vi "GetTests.vi"(8 "error in (no error)":errorcluster, 11 "reference in":refnum<class "MES_Local.lvclass">) -> (0 "error out":errorcluster, 1 "Active Test Index":i32, 2 "Tests":T1[](array[typedef]), 3 "reference in":refnum<class "MES_Local.lvclass">)   [LabVIEW 2022 SP3, in "MES_Local.lvlib" / "MES_Local.lvclass"]
uses:
  MES_Local.lvclass
  Components/MES_Base.lvlibp/Controls/Test.ctl
  Components/MES_Base.lvlibp/MES_Base.lvclass
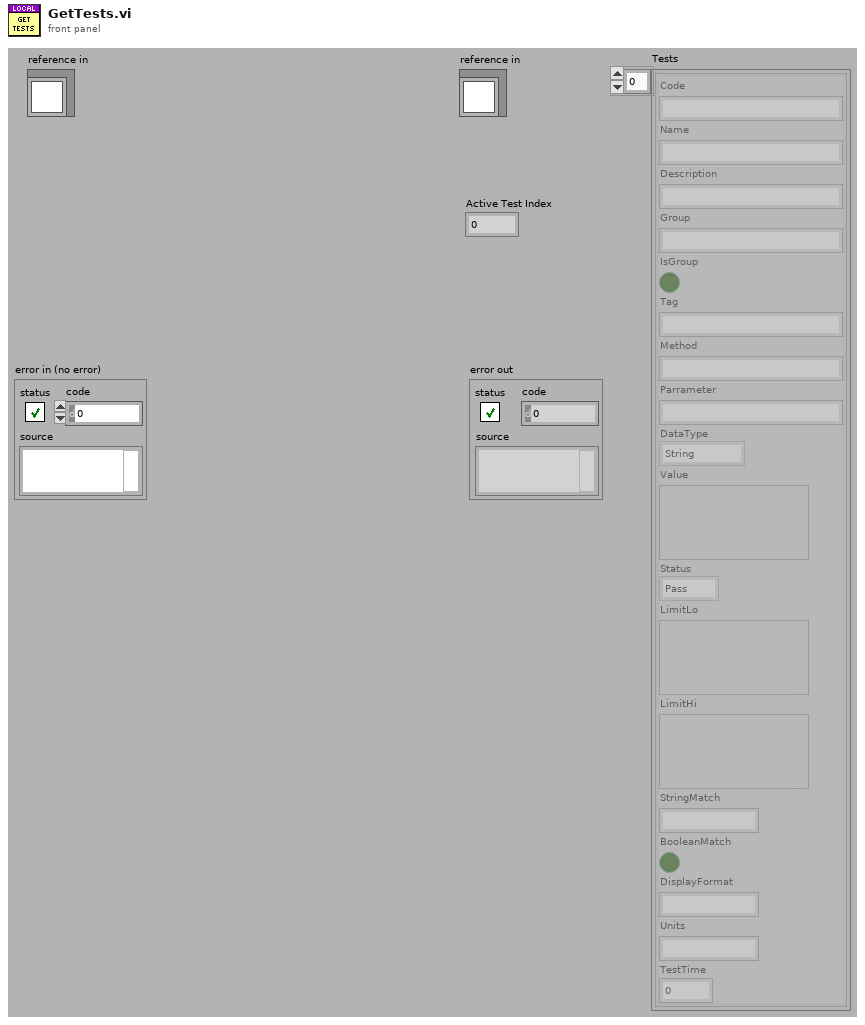
[diagram p1: front panel]
types:
  T1 = typedef "MES_Base.lvlibp/MES_Base.lvclass/Test.ctl" = cluster{"Code":string, "Name":string, "Description":string, "Group":string, "IsGroup":bool, "Tag":string, "Method":string, "Parrameter":string, "DataType":enum16{"NA", "String", "Boolean", "Int", "Dbl"}, "Value":variant, "Status":enum16{"Pending", "Pass", "Fail"}, "LimitLo":variant, "LimitHi":variant, "StringMatch":string, "BooleanMatch":bool, "DisplayFormat":string, "Units":string, "TestTime":dbl}
  T2 = typedef "MES_Local.lvlib/MES_Local.lvclass/ObjectAttributes.ctl" = cluster{"Config":T3, "Logged_In?":bool, "AttributeNames":string[], "AttributeWritten":bool[], "ComponentNames":string[], "TestIndex":i32, "TestTag":string[], "Time Stamp":timestamp, "Employee":string, "Resource_Key":string, "Local Spec":path, "Login":refnum<class "Login_Base.lvclass">, "ReportPath":path, "Spec":T4, "StartTime":timestamp, "Role":string}
  T3 = typedef "MES_Local.lvlib/MES_Local.lvclass/Config.ctl" = cluster{"Results_Path":path}
  T4 = typedef "MES_Base.lvlibp/MES_Base.lvclass/Spec.ctl" = cluster{"Header":cluster{"Doctype":string, "Checksum":string, "DriverKey":string, "SpecId":string, "TransactionId":string, "AccountId":string, "SpecName":string, "WorkflowStep":string, "SerialNumber":string, "BatchNumber":string, "Status":enum16{"Pending", "Pass", "Fail"}, "Comment":string, "FirstFail":string, "Employee":string, "LocalMachine":string, "ResourceKey":string, "Date":string, "Time":string, "Duration":string, "DUT Position":i32}, "Components":cluster{"SerialNumber":string, "PartNumber":string, "Revision":string, "BatchNumber":string, "Name":string, "Description":string, "Attached":bool}[], "Attributes":cluster{"Name":string, "Description":string, "DataType":enum16{"NA", "String", "Boolean", "Int", "Dbl"}, "Value":variant, "DisplayFormat":string, "ReadOnly":bool, "Required":bool}[], "Tests":cluster{"Code":string, "Name":string, "Description":string, "Group":string, "IsGroup":bool, "Tag":string, "Method":string, "Parrameter":string, "DataType":enum16{"NA", "String", "Boolean", "Int", "Dbl"}, "Value":variant, "Status":enum16{"Pending", "Pass", "Fail"}, "LimitLo":variant, "LimitHi":variant, "StringMatch":string, "BooleanMatch":bool, "DisplayFormat":string, "Units":string, "TestTime":dbl}[]}
  T5 = cluster{"Code":string, "Name":string, "Description":string, "Group":string, "IsGroup":bool, "Tag":string, "Method":string, "Parrameter":string, "DataType":enum16{"NA", "String", "Boolean", "Int", "Dbl"}, "Value":variant, "Status":enum16{"Pending", "Pass", "Fail"}, "LimitLo":variant, "LimitHi":variant, "StringMatch":string, "BooleanMatch":bool, "DisplayFormat":string, "Units":string, "TestTime":dbl}[]
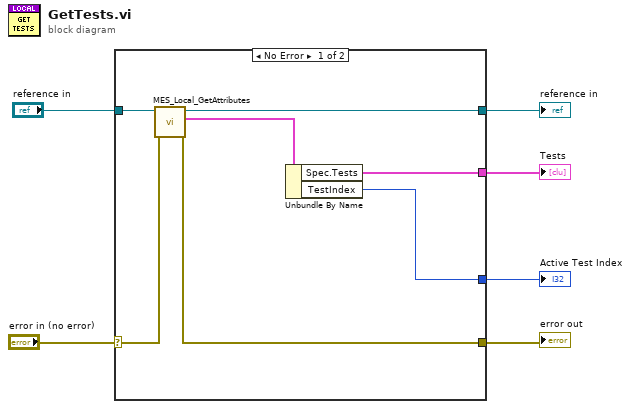
[diagram p0: block diagram]
diagram:
  n1 = case shown="No Error" "error in (no error)" {
    selector: "error in (no error)" -> [w13 w15]
    tunnel: [w11 w15] -> w5
    tunnel: [w9 w14] -> w3
    tunnel: "reference in" -> [w10 w14]
    tunnel: [w8 _] -> w2
    tunnel: [w7 _] -> w1
    frame No Error {
      n2 = call "MES_Local_GetAttributes.vi"("error in (no error)"=w13, "reference in"=w10) -> ("error out"=w11:errorcluster, "Data"=w12:T2, "reference out"=w9:refnum<class "MES_Local.lvclass">)  [unwired: 6 in, 1 out]
      n3 = Unbundle By Name(w12) -> ("Spec.Tests"=w8:T5, "TestIndex"=w7:i32)
    }
    frame Error {
    }
  }
  "error out" <- w5
  "reference in" <- w3
  "Active Test Index" <- w1
  "Tests" <- w2
